vi "SubPanelTypecast.vi"(0 "Ctl Refnum":refnum<vi>, 7 "Control Path In":string[](array[string]), 11 "Error In":errorcluster) -> (4 "Controls[]":refnum<vi>[](array[refnum]), 8 "Control Path Out":string[](array[string]), 15 "Error Out":errorcluster)   [LabVIEW 2016, in "Drona.lvlib" / "GetControlRef.lvlib"]
doc: "Gives the reference of controls present inside the inserted VI of the SubPanel"
uses:
  GetControlRef.lvlib
  Drona.lvlib
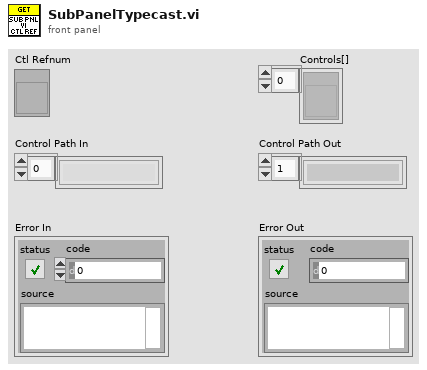
[diagram p1: front panel]
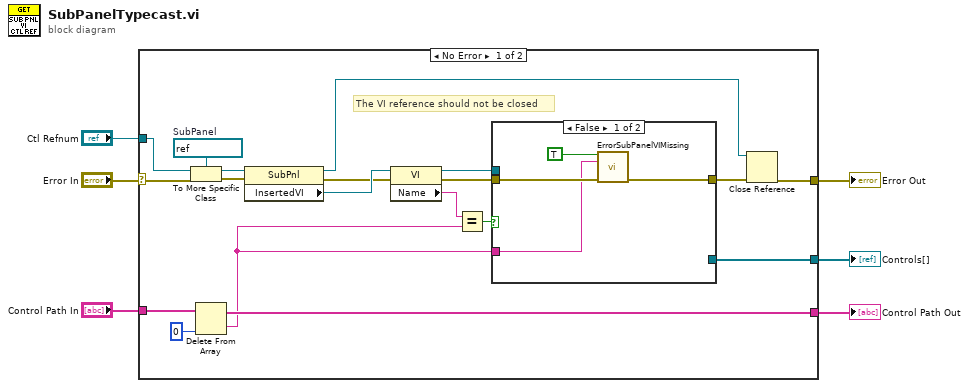
[diagram p0: block diagram]
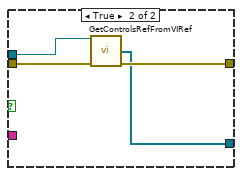
[diagram p2: hidden frame]
diagram:
  n1 = case shown="No Error" "Error In" {
    selector: "Error In" -> [w13 w35]
    tunnel: "Control Path In" -> [w25 w34]
    tunnel: "Ctl Refnum" -> [w24 _]
    tunnel: [w16 _] -> w4
    tunnel: [w15 w34] -> w3
    tunnel: [w14 w35] -> w2
    frame No Error {
      w21 = refnum<vi> refnum  # SubPanel
      # "The VI reference should not be closed"
      n2 = To More Specific Class(target class=w21, reference=w24, error in=w13) -> (specific class reference=w23:refnum<vi>, error out=w22:errorcluster)
      n3 = Delete From Array(array=w25, index=0) -> (deleted portion=w7:string, array with subset deleted=w15:string[])  [unwired: 1 in]
      n4 = property class="SubPnl"(reference=w23, error in=w22) -> (reference out=w18:refnum<vi>, error out=w19:errorcluster, "InsertedVI"=w20:refnum<vi>)
      n5 = property class="VI"(reference=w20, error in=w19) -> (reference out=w9:refnum<vi>, error out=w10:errorcluster, "Name"=w12:string)
      n6 = Equal?(x=w12, y=w7) -> (x = y?=w11:bool)
      n7 = case shown="False" w11 {
        tunnel: w10 -> [w29 w32]
        tunnel: [w28 w31] -> w8
        tunnel: w9 -> [_ w33]
        tunnel: [_ w30] -> w16
        tunnel: w7 -> [w27 _]
        frame False {
          n8 = call "ErrorSubPanelVIMissing.vi"("Create Error?"=TRUE, "VI Name"=w27, "error in"=w29) -> ("error out"=w28:errorcluster)  [unwired: 12 in]
        }
        frame True {
          n9 = call "GetControlsRefFromVIRef.vi"("VI Reference In"=w33, "Error In"=w32) -> ("Controls[]"=w30:refnum<vi>[], "Error Out"=w31:errorcluster)  [unwired: 11 in, 1 out]
        }
      }
      n10 = Close Reference(reference=w18, error in (no error)=w8) -> (error out=w14:errorcluster)
    }
    frame Error {
    }
  }
  "Controls[]" <- w4
  "Control Path Out" <- w3
  "Error Out" <- w2
